vi "macro_LinearSystemLoop_LinearSystem_Execute.vi"() -> ()   [LabVIEW 2019, in "Trajectory_Library.lvlib"]
uses:
  Trajectory_Library.lvlib
  <vilib>/Analysis/Matrix/Datatypes/RealMatrix.ctl
  MatrixHelper_CoerceSize.vi
  MatBuilder_Create.vi
  <vilib>/Analysis/Matrix/NI_Matrix.lvlib
panel:
  in  "ProcessVariables":dbl[](array[numeric])
  in  "Setpoints":dbl[](array[numeric])
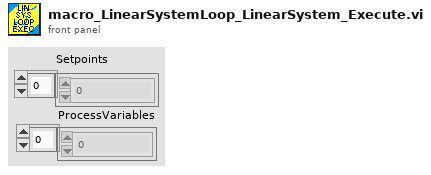
[diagram p1: front panel]
types:
  T1 = typedef "NI_Matrix.lvlib/RealMatrix.ctl" = dbl[][]
  T2 = typedef "Trajectory_Library.lvlib/LINEAR_SYSTEM.ctl" = cluster{"m_A":T1, "m_B":T1, "m_C":T1, "m_D":T1, "States":i32, "Inputs":i32, "Outputs":i32}
  T3 = typedef "Trajectory_Library.lvlib/LINEAR_SYSTEM_LOOP_CTRL_PARAMS.CTL" = cluster{"Model Std Dev":dbl[], "Measure Std Dev":dbl[], "Control Tol":dbl[], "Max Control Effort":dbl[]}
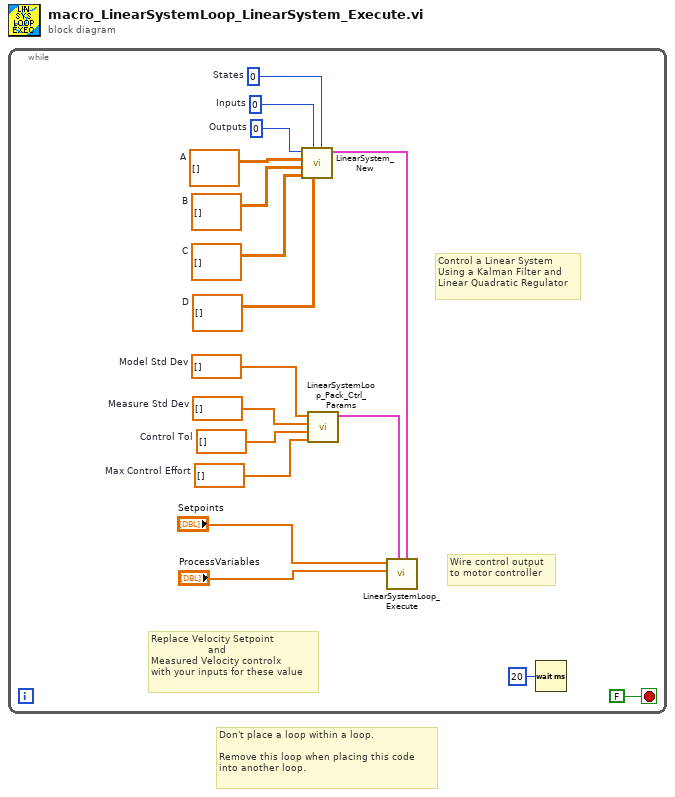
[diagram p0: block diagram]
diagram:
  # "Don't place a loop within a loop.\n \nRemove this loop when placing this code\ninto another loop."
  n1 = while {
    stop <- FALSE stop-if-true
    w1 = 0  # Outputs
    w2 = T1 []  # A
    w3 = T1 []  # B
    w4 = T1 []  # C
    w5 = T1 []  # D
    w6 = 0  # States
    w7 = 0  # Inputs
    w11 = dbl[] []  # Model Std Dev
    w12 = dbl[] []  # Measure Std Dev
    w13 = dbl[] []  # Control Tol
    w14 = dbl[] []  # Max Control Effort
    # "Wire control output\nto motor controller"
    # "Replace Velocity Setpoint \n                   and \nMeasured Velocity controlx\nwith your inputs for these value"
    # "Control a Linear System\nUsing a Kalman Filter and \nLinear Quadratic Regulator"
    n2 = call "LinearSystem_New.vi"("States"=w6, "D"=w5, "Inputs"=w7, "C"=w4, "B"=w3, "A"=w2, "Outputs"=w1) -> ("Linearsystem"=w10:T2)  [unwired: 3 in, 1 out]
    n3 = call "LinearSystemLoop_Pack_Ctrl_Params.vi"("Max Control Effort"=w14, "Control Tol"=w13, "Measure Std Dev"=w12, "Model Std Dev"=w11) -> ("LinearSystemLoop_Control_Params"=w15:T3)  [unwired: 7 in]
    n4 = call "LinearSystemLoop_Execute.vi"("Linear System"=w10, "LinearSystemLoop_Control_Params"=w15, "ProcessVariables"="ProcessVariables", "Setpoints"="Setpoints") -> ()  [unwired: 4 in, 4 out]
    n5 = Wait (ms)(milliseconds to wait=u32 20) -> ()  [unwired: 1 out]
  }
